vi "poly_trim(m)_xwav(m).vi"(8 "Error in":errorcluster caption="Error in (no error)", 9 "end x's":dbl[](array[numeric]), 10 "start x's":dbl[](array[numeric]), 11 "array of xwavs in":T1[](array[typedef])) -> (0 "Error out":errorcluster, 1 "actual end x's":dbl[](array[numeric]) format="%0.2f", 2 "actual start x's":dbl[](array[numeric]) format="%0.2f", 3 "array of xwavs out":T1[](array[typedef]))   [LabVIEW 2015, in "_xwav_polys.lvlib"]
uses:
  _xwav_polys.lvlib
  xwav.ctl
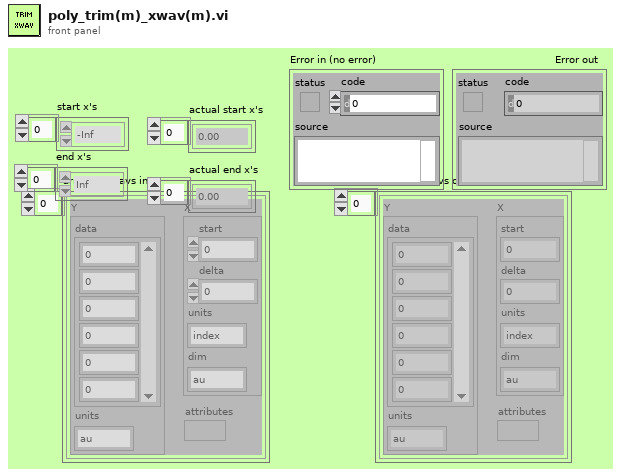
[diagram p1: front panel]
types:
  T1 = typedef "xwav.ctl" = cluster{"attributes":variant, "X":cluster{"start":dbl, "delta":dbl, "units":string, "dim":string}, "Y":cluster{"data":dbl[], "units":string}}
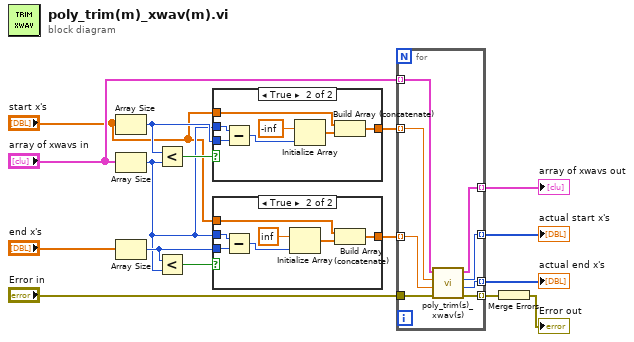
[diagram p0: block diagram]
diagram:
  n1 = Array Size(array="start x's") -> (size(s)=w12:i32)
  n2 = Array Size(array="array of xwavs in") -> (size(s)=w10:i32)
  n3 = Array Size(array="end x's") -> (size(s)=w11:i32)
  n4 = Less?(x=w12, y=w10) -> (x < y?=w13:bool)
  n5 = Less?(x=w11, y=w10) -> (x < y?=w5:bool)
  n6 = case shown="True" w13 {
    tunnel: "start x's" -> [w17 w20]
    tunnel: w10 -> [_ w23]
    tunnel: w12 -> [_ w22]
    tunnel: [w17 w18] -> w9
    frame False {
    }
    frame True {
      n7 = Subtract(x=w23, y=w22) -> (x-y=w21:i32)
      n8 = Initialize Array(-inf ("element"), w21) -> (w19:dbl[])
      n9 = Build Array (concatenate)(w20, w19) -> (w18:dbl[])
    }
  }
  n10 = case shown="True" w5 {
    tunnel: w10 -> [_ w31]
    tunnel: w11 -> [_ w30]
    tunnel: [w25 w27] -> w8
    tunnel: "start x's" -> [w25 w26]
    frame False {
    }
    frame True {
      n11 = Subtract(x=w31, y=w30) -> (x-y=w29:i32)
      n12 = Initialize Array(inf ("element"), w29) -> (w28:dbl[])
      n13 = Build Array (concatenate)(w26, w28) -> (w27:dbl[])
    }
  }
  n14 = for {
    tunnel: [w40] -> w7 mode=indexing
    tunnel: [w39] -> w6 mode=indexing
    tunnel: "array of xwavs in" -> [w38] mode=indexing
    tunnel: [w37] -> w16 mode=indexing
    tunnel: w9 -> [w36] mode=indexing
    tunnel: w8 -> [w35] mode=indexing
    tunnel: "Error in" -> [w34]
    tunnel: [w33] -> w2 mode=indexing
    n15 = call "poly_trim(s)_xwav(s).vi"("Error in"=w34, "end x (end)"=w35, "start x (start)"=w36, "xwave in"=w38) -> ("Error out"=w33:errorcluster, "actual end x index"=w39:i32, "actual start x index"=w40:i32, "xwave out"=w37:T1)  [unwired: 4 in]
  }
  "array of xwavs out" <- w16
  "actual start x's" <- w7
  "actual end x's" <- w6
  n16 = Merge Errors(w2) -> (→"Error out":errorcluster)
